vi "Create_directory_option.vi"(0 "Filename":path) -> (1 "Path is to existing File":bool, 2 "Path is to existing Directory":bool)   [LabVIEW 2010]
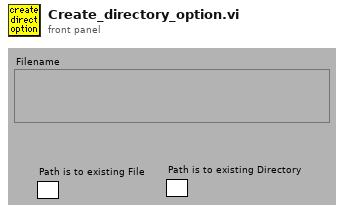
[diagram p1: front panel]
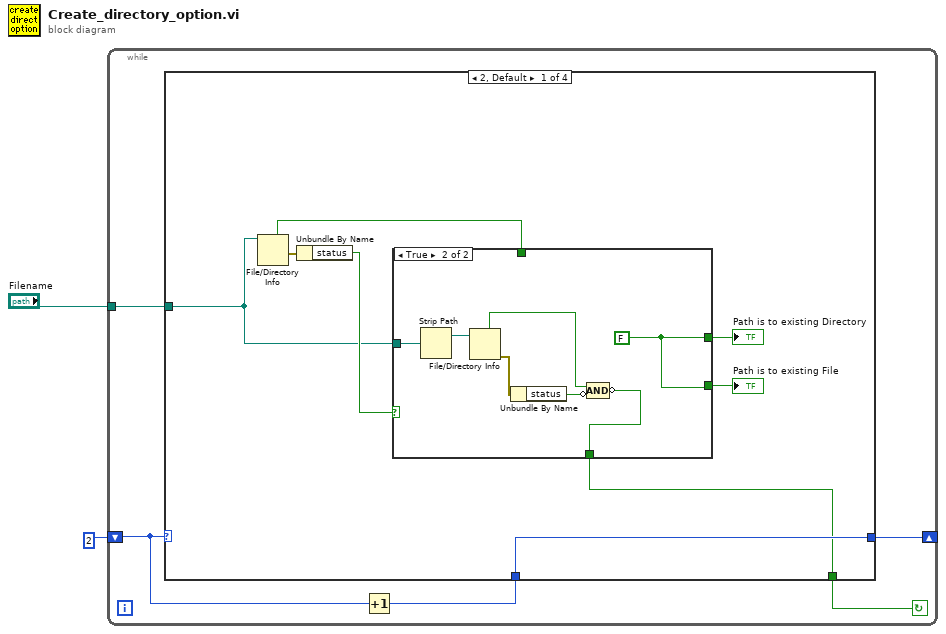
[diagram p0: block diagram]
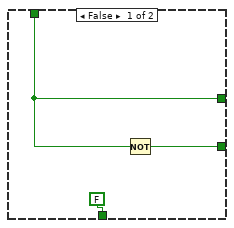
[diagram p2: hidden frame]
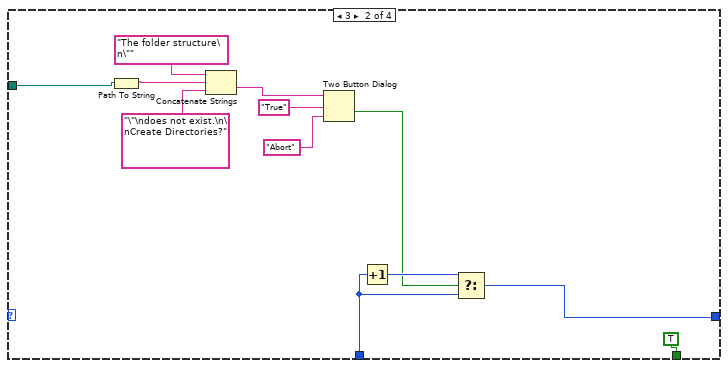
[diagram p3: hidden frame]
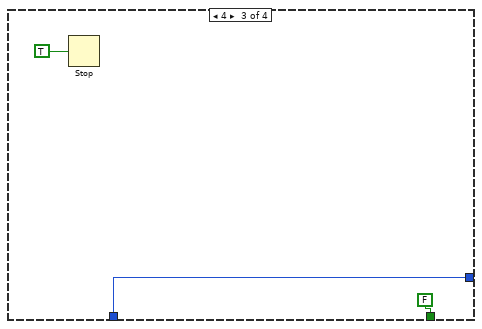
[diagram p4: hidden frame]
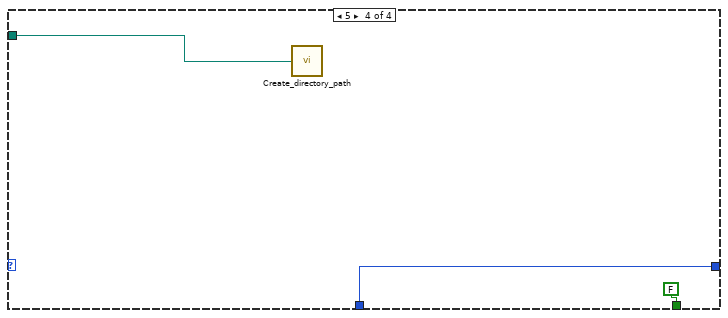
[diagram p5: hidden frame]
diagram:
  n1 = while {
    tunnel: "Filename" -> [w3]
    shift-left: 2 -> [w6]
    shift-right: [w4] -> _
    stop <- w7 continue-if-true
    n2 = Increment(x=w6) -> (x+1=w5:i32)
    n3 = case shown="2, Default" w6 {
      tunnel: [w8 TRUE ("status") FALSE ("status") FALSE ("status")] -> w7
      tunnel: w5 -> [w15 w29 w38 w43]
      tunnel: [w15 w27 w38 w43] -> w4
      tunnel: w3 -> [w9 w31 _ w41]
      frame 2, Default {
        n4 = File/Directory Info(path=w9) -> (directory=w11:bool, error out=w14:errorcluster)  [unwired: 1 in, 5 out]
        n5 = Unbundle By Name(w14) -> ("status"=w10:bool)
        n6 = case shown="True" w10 {
          tunnel: [w18 w22] -> w13
          tunnel: [w17 w22] -> w12
          tunnel: w11 -> [w18 _]
          tunnel: w9 -> [_ w24]
          tunnel: [FALSE ("status") w19] -> w8
          frame False {
            n7 = Not(x=w18) -> (.not. x?=w17:bool)
          }
          frame True {
            w22 = FALSE ("Directory exists")
            n8 = Strip Path(path=w24) -> (stripped path=w23:path)  [unwired: 1 out]
            n9 = File/Directory Info(path=w23) -> (directory=w21:bool, error out=w25:errorcluster)  [unwired: 1 in, 5 out]
            n10 = Unbundle By Name(w25) -> ("status"=w20:bool)
            n11 = Compound Arithmetic op=AND(w21, invert w20) -> (invert w19:bool)
          }
        }
        "Path is to existing File" <- w12
        "Path is to existing Directory" <- w13
      }
      frame 3 {
        n12 = Path To String(path=w31) -> (string=w37:string)
        n13 = Concatenate Strings("The folder structure\n\"", w37, "\"\ndoes not exist.\n\nCreate Directories?") -> (w34:string)
        n14 = Two Button Dialog(message=w34, 1:"Abort" ("F button name (\"Cancel\")"), 2:"True" ("T button name (\"OK\")")) -> (T button?=w26:bool)
        n15 = Increment(x=w29) -> (x+1=w28:i32)
        n16 = Select(t=w28, s=w26, f=w29) -> (s? t:f=w27:i32)
      }
      frame 4 {
        n17 = Stop(stop? (T)=TRUE) -> ()
      }
      frame 5 {
        n18 = call "Create_directory_path.vi"("Path name"=w41) -> ()  [unwired: 1 out]
      }
    }
  }
